vi "Detector_setup.vi"(0 "Select Detector":enum8{"CCD-1024x256", "InGaAs PDA-1024x1"}(ring), 5 "error in":errorcluster) -> (8 "error out":errorcluster)   [LabVIEW 2024]
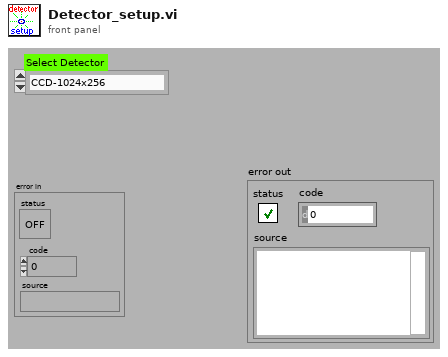
[diagram p1: front panel]
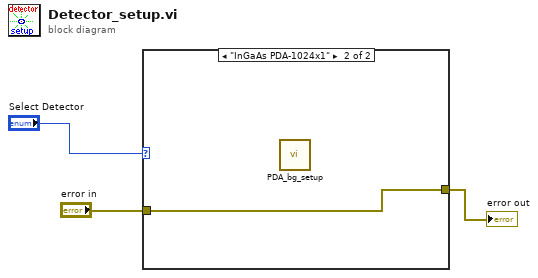
[diagram p0: block diagram]
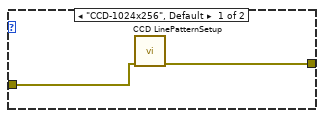
[diagram p2: hidden frame]
diagram:
  n1 = case shown="\"InGaAs PDA-1024x1\"" "Select Detector" {
    tunnel: "error in" -> [w5 w6]
    tunnel: [w4 w6] -> w1
    frame "CCD-1024x256", Default {
      n2 = call "CCD LinePatternSetup.vi"("error in"=w5) -> ("error out"=w4:errorcluster)  [unwired: 7 in, 2 out]
    }
    frame "InGaAs PDA-1024x1" {
      n3 = call "PDA_bg_setup.vi"() -> ()  [unwired: 1 in]
    }
  }
  "error out" <- w1
